vi "_BlankServer.vi"() -> ()   [LabVIEW 2012]
uses:
  ServerSubs/MyState.ctl
  ServerSubs/ROSLog.ctl
  SubVIs/_ROSDirection.ctl
  SubVIs/_ROSControl.ctl
  ServerSubs/requestTopic.ctl
panel:
  out "Log of port":string
  out "Queue log":string
  out "Last Reply":string
  out "Registered topics":T1[](array[typedef])
  out "Registering":bool
  out "MyState":T3
  out "(Un)Reg Text":string
  out "Setup":string
  out "Cmd Log":T4[](array[typedef])
  out "Connections Error log":string
  out "Connections":T5(array[cluster])
  out "Error log":string
  in  "stop":bool
  in  "ROS":T1={"topic port"=1236, "Node"="/labview", "topic"="/robot/head/command_head_nod", "type"="std_msgs/Bool", "node port"=7000, "error "={"status"=FALSE, "code"=0, "source"=""}, "Direction"=enum."Publisher", "APIs"=[], "Update (ms)"=1, "write queue"=1}
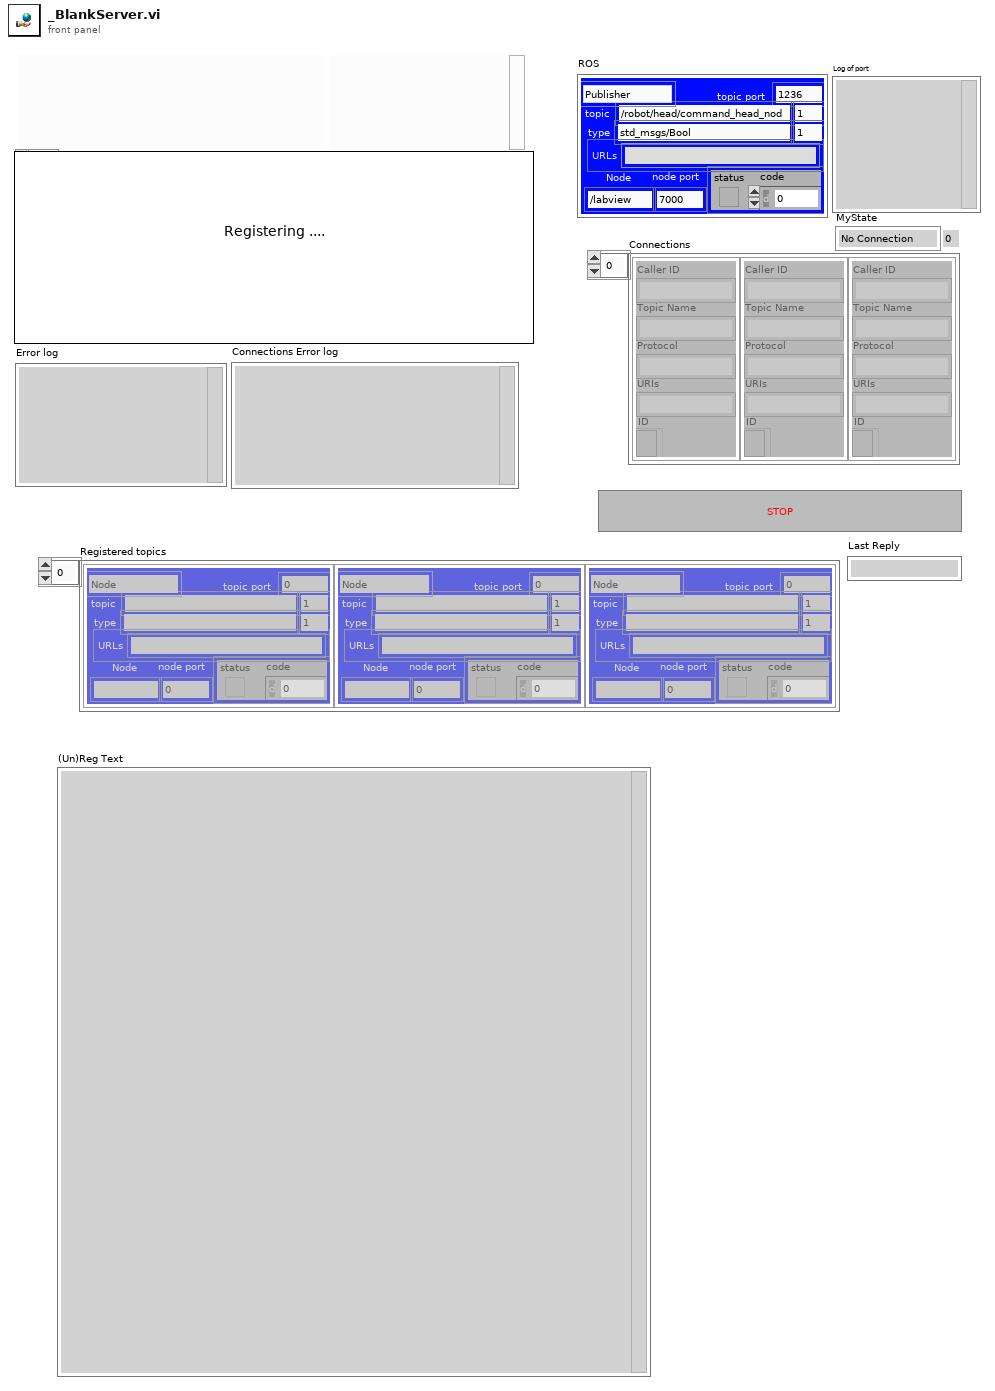
[diagram p1: front panel]
types:
  T1 = typedef "_ROSControl.ctl" = cluster{"topic port":u16, "Node":string, "topic":string, "type":string, "node port":u32, "error ":errorcluster, "Direction":T2, "APIs":string[], "Update (ms)":u16, "write queue":u16}
  T2 = typedef "_ROSDirection.ctl" = enum16{"Node", "Publisher", "Subscriber", "Service Client"}
  T3 = typedef "MyState.ctl" = enum16{"No Connection", "Registered", "Connected", "Close"}
  T4 = typedef "ROSLog.ctl" = cluster{"Sent":string, "Reply":string, "MethodName":string, "success":bool, "Dir1":string, "Dir2":string, "Time Stamp":string}
  T5 = cluster{"Caller ID":string, "Topic Name":string, "Protocol":string, "URIs":string, "ID":refnum<k5>}[]
  T6 = typedef "requestTopic.ctl" = cluster{"New Subscriber":cluster{"Caller ID":string, "Topic Name":string, "Protocol":string, "URIs":string, "ID":refnum<k5>}, "ROS of Server":T1, "new port":u16}
  T7 = cluster{"Code":i32, "Status Message":string, "APIs":string[]}
  T8 = cluster{"Caller ID":string, "Topic Name":string, "Protocol":string, "URIs":string, "ID":refnum<k5>}
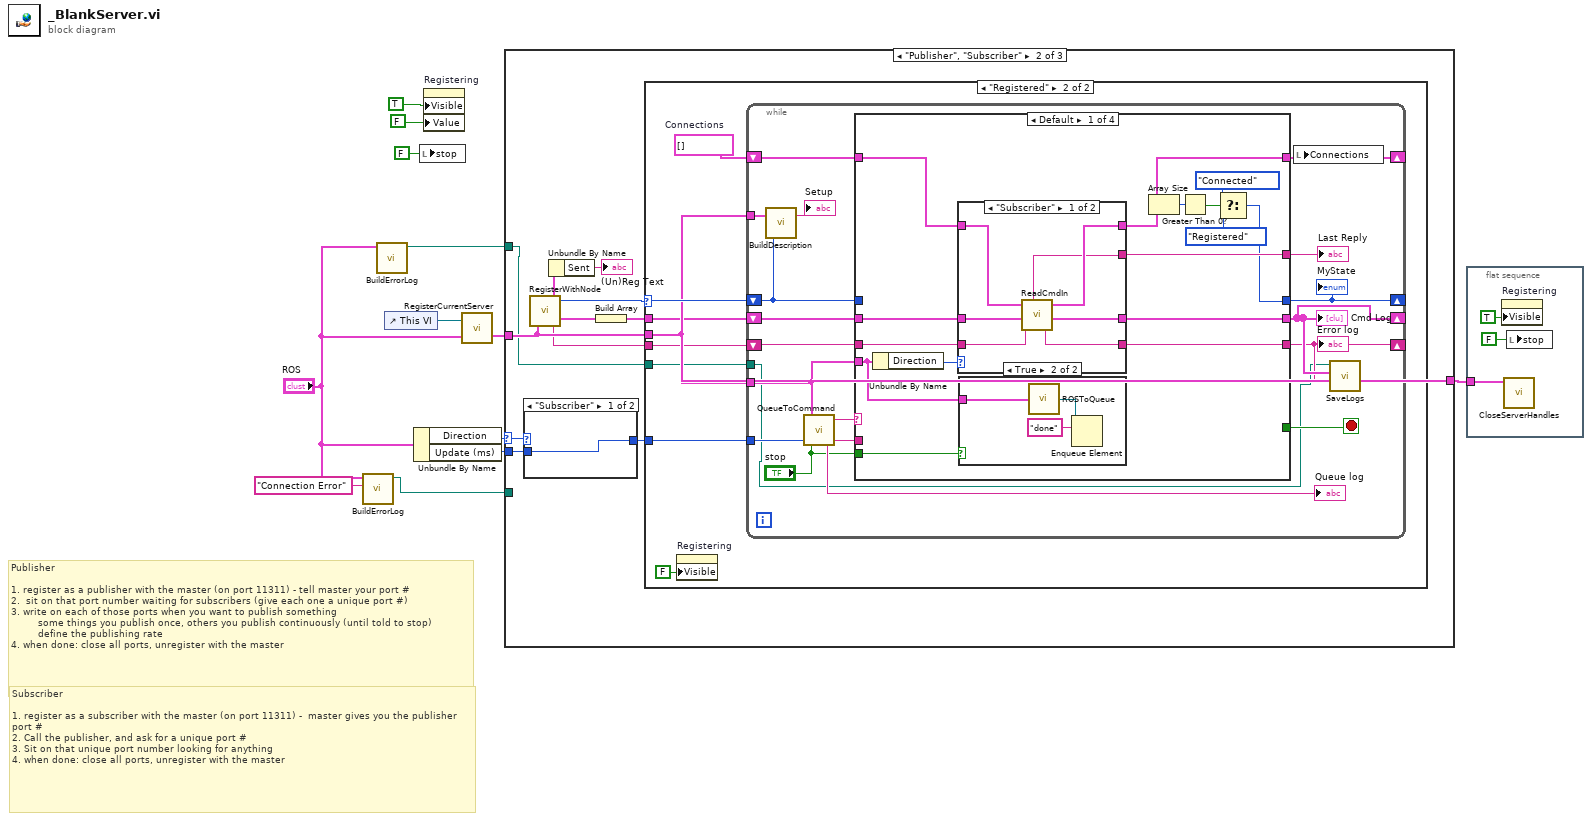
[diagram p0: block diagram]
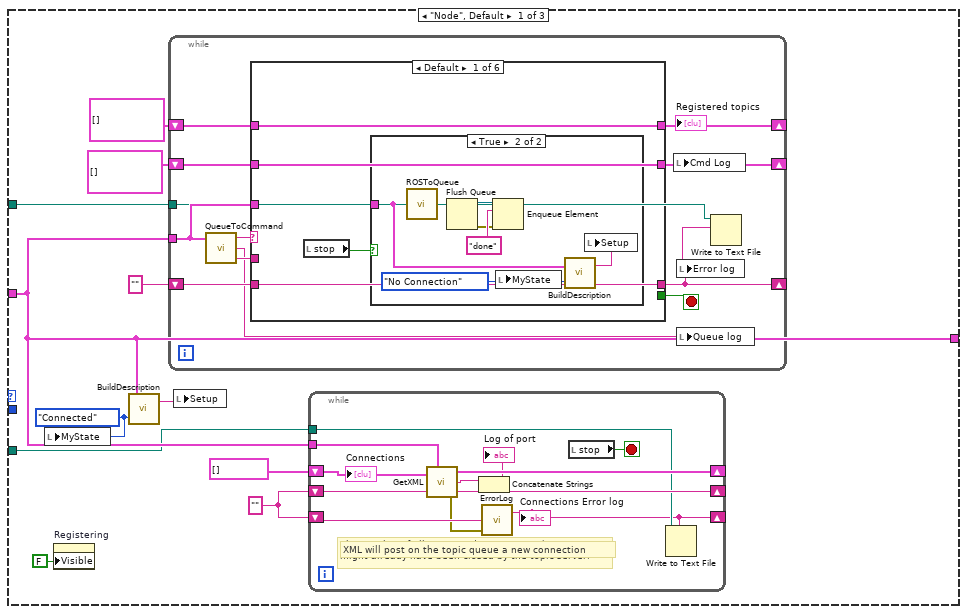
[diagram p2: hidden frame]
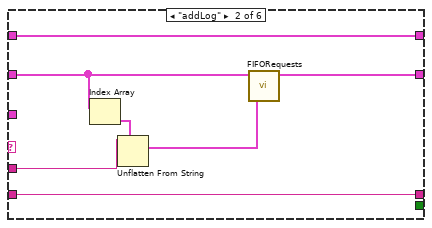
[diagram p4: hidden frame]
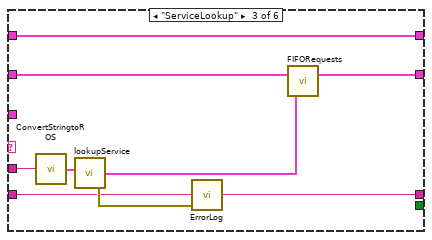
[diagram p5: hidden frame]
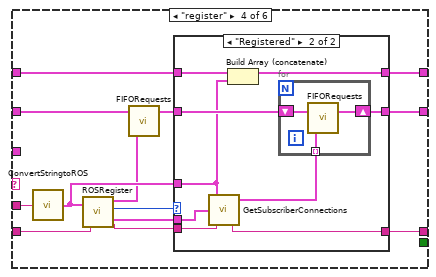
[diagram p6: hidden frame]
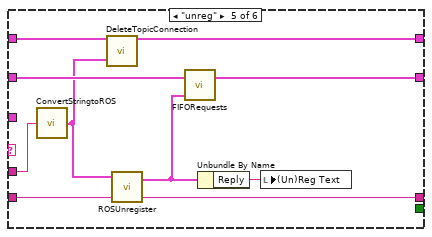
[diagram p8: hidden frame]
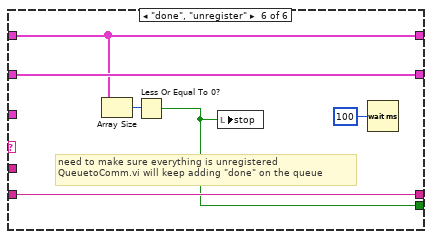
[diagram p9: hidden frame]
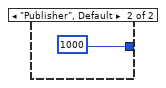
[diagram p10: hidden frame]
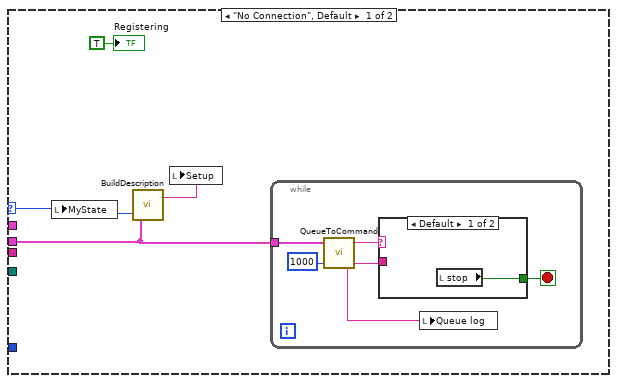
[diagram p11: hidden frame]
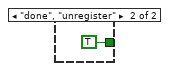
[diagram p12: hidden frame]
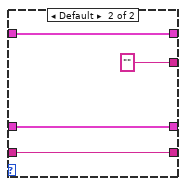
[diagram p13: hidden frame]
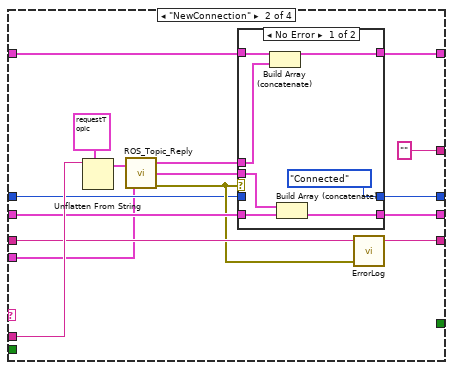
[diagram p15: hidden frame]
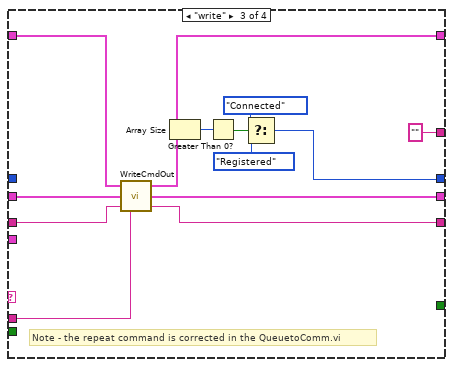
[diagram p17: hidden frame]
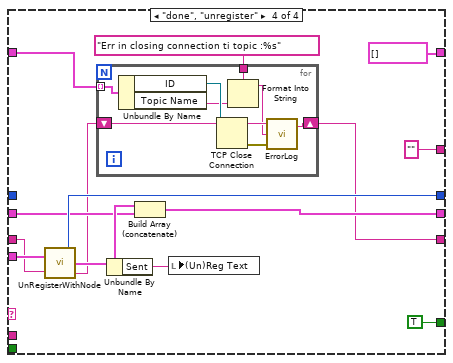
[diagram p18: hidden frame]
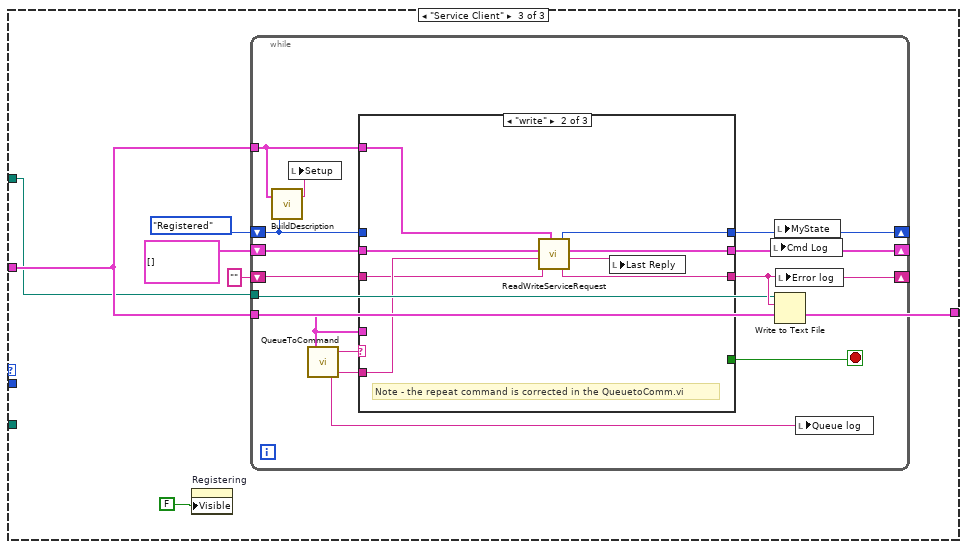
[diagram p19: hidden frame]
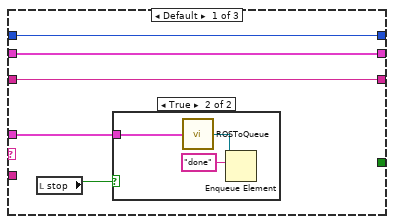
[diagram p20: hidden frame]
diagram:
  # "Subscriber\n\n1. register as a subscriber with the master (on port 11311) -  master gives you the publisher port #\n2. Call the publisher, and ask for a unique port #\n3. Sit on that unique port number looking for anything\n4. when done: close all ports, unregister with the master"
  # "Publisher\n\n1. register as a publisher with the master (on port 11311) - tell master your port #\n2.  sit on that port number waiting for subscribers (give each one a unique port #)\n3. write on each of those ports when you want to publish something\n         some things you publish once, others you publish continuously (until told to stop)\n         define the publishing rate\n4. when done: close all ports, unregister with the master"
  n1 = call "BuildErrorLog.vi"("Error Type"="Connection Error", "ROS"="ROS") -> ("error log path"=w1:path)  [unwired: 9 in]
  n2 = call "BuildErrorLog.vi"("ROS"="ROS") -> ("error log path"=w4:path)  [unwired: 10 in]
  n3 = control-ref of="This VI"() -> (w7:refnum<vi>)
  n4 = Unbundle By Name("ROS") -> ("Direction"=w10:T2, "Update (ms)"=w5:u16)
  n5 = local write "stop"(FALSE ("stop")) -> ()
  n6 = property on="Registering" class="Bool (strict)"("Visible"=TRUE ("Registering"), "Value"=FALSE ("Registering")) -> ()  [unwired: 2 in, 2 out]
  n7 = call "RegisterCurrentServer.vi"("ROS in"="ROS", "This VI"=w7) -> ("ROS out"=w6:T1)  [unwired: 1 in]
  n8 = case shown="\"Publisher\", \"Subscriber\"" w10 {
    selector: w10 -> [_ w125 _]
    tunnel: w6 -> [w17 w128 w265]
    tunnel: [w17 w128 w265] -> w8
    tunnel: w5 -> [_ w120 _]
    tunnel: w4 -> [w14 w119 w260]
    tunnel: w1 -> [w13 _ _]
    frame "Node", Default {
      w16 = "" ("String out")
      w21 = MyState."Connected" ("MyState")
      n9 = local write "MyState"(w21) -> ()
      n10 = property on="Registering" class="Bool (strict)"("Visible"=FALSE ("Registering")) -> ()  [unwired: 2 in, 2 out]
      n11 = call "BuildDescription.vi"("MyState"=w21, "ROS in"=w17) -> ("Setup"=w22:string)  [unwired: 1 in]
      n12 = while {
        shift-right: [w25] -> _
        shift-left: "" ("String out") -> [w34]
        shift-right: [w33] -> _
        shift-left: T4[] [] ("Requests Out") -> [w32]
        shift-right: [w31] -> _
        shift-left: T1[] [] -> [w30]
        tunnel: w17 -> [w26]
        tunnel: w14 -> [w24]
        stop <- w35 stop-if-true
        n13 = call "QueueToCommand.vi"("ROS"=w26) -> ("data"=w28:string, "Queue log"=w27:string, "Command"=w29:string)  [unwired: 2 in]
        n14 = case shown="Default" w29 {
          tunnel: [_ _ _ _ _ w103] -> w35
          tunnel: w28 -> [_ w52 w62 w76 w101 _]
          tunnel: w34 -> [w40 w54 w59 w75 w100 w107]
          tunnel: [w40 w54 w58 w64 w99 w107] -> w25
          tunnel: [w39 w48 w55 w74 w96 w106] -> w33
          tunnel: w32 -> [w39 w49 w56 w67 w97 w106]
          tunnel: [w38 w53 w63 w72 w93 w105] -> w31
          tunnel: w30 -> [w38 w53 w63 w73 w94 w105]
          tunnel: w26 -> [w36 _ _ _ _ _]
          frame Default {
            n15 = local read "stop"() -> (w37:bool)
            n16 = case shown="True" w37 {
              tunnel: w36 -> [_ w42]
              frame False {
              }
              frame True {
                w43 = MyState."No Connection" ("MyState")
                n17 = call "ROSToQueue.vi"("ROS"=w42) -> ("queue"=w45:refnum<queue>)  [unwired: 3 in, 1 out]
                n18 = Flush Queue(queue=w45) -> (queue out=w41:refnum<queue>, error out=w46:errorcluster)  [unwired: 1 in, 1 out]
                n19 = Enqueue Element(queue=w41, element="done" ("regular expression"), error in (no error)=w46) -> ()  [unwired: 1 in, 3 out]
                n20 = local write "MyState"(w43) -> ()
                n21 = call "BuildDescription.vi"("MyState"=w43, "ROS in"=w42) -> ("Setup"=w44:string)  [unwired: 1 in]
                n22 = local write "Setup"(w44) -> ()
              }
            }
          }
          frame "addLog" {
            n23 = Index Array(array=w49) -> (element=w51:T4)  [unwired: 1 in]
            n24 = Unflatten From String(type=w51, binary string=w52) -> (value=w50:T4)  [unwired: 3 in, 2 out]
            n25 = call "FIFORequests.vi"("Log"=w50, "Requests in"=w49) -> ("Requests out"=w48:T4[])  [unwired: 1 in]
          }
          frame "ServiceLookup" {
            n26 = call "ConvertStringtoROS.vi"("string in"=w62) -> ("ROS"=w61:T1)
            n27 = call "lookupService.vi"("Service ROS"=w61) -> ("error out"=w60:errorcluster, "Log"=w57:T4)  [unwired: 3 in]
            n28 = call "ErrorLog.vi"("error in"=w60, "String in"=w59) -> ("String out"=w58:string)  [unwired: 1 in, 1 out]
            n29 = call "FIFORequests.vi"("Log"=w57, "Requests in"=w56) -> ("Requests out"=w55:T4[])  [unwired: 1 in]
          }
          frame "register" {
            n30 = call "ConvertStringtoROS.vi"("string in"=w76) -> ("ROS"=w71:T1)
            n31 = call "ROSRegister.vi"("Err In"=w75, "ROS to register"=w71) -> ("Err Out"=w65:string, "Response"=w70:T7, "MyState"=w69:T3, "Log"=w68:T4)
            n32 = call "FIFORequests.vi"("Log"=w68, "Requests in"=w67) -> ("Requests out"=w66:T4[])  [unwired: 1 in]
            n33 = case shown="\"Registered\"" w69 {
              tunnel: w66 -> [w78 w88]
              tunnel: [w78 w87] -> w74
              tunnel: w73 -> [w79 w86]
              tunnel: [w79 w85] -> w72
              tunnel: w71 -> [_ w83]
              tunnel: w70 -> [_ w82]
              tunnel: w65 -> [w77 w81]
              tunnel: [w77 w80] -> w64
              frame Default {
              }
              frame "Registered" {
                n34 = call "GetSubscriberConnections.vi"("Err in"=w81, "Response"=w82, "ROS registered"=w83) -> ("Err out"=w80:string, "Logs out"=w84:T4[])  [unwired: 1 out]
                n35 = Build Array (concatenate)(w86, w83) -> (w85:T1[])
                n36 = for {
                  tunnel: w84 -> [w89] mode=indexing
                  shift-right: [w90] -> w87
                  shift-left: w88 -> [w91]
                  n37 = call "FIFORequests.vi"("Log"=w89, "Requests in"=w91) -> ("Requests out"=w90:T4[])  [unwired: 1 in]
                }
              }
            }
          }
          frame "unreg" {
            n38 = call "ConvertStringtoROS.vi"("string in"=w101) -> ("ROS"=w92:T1)
            n39 = call "DeleteTopicConnection.vi"("ROS"=w92, "Con In"=w94) -> ("Con out"=w93:T1[])
            n40 = call "ROSUnregister.vi"("Err in"=w100, "Server ROS"=w92) -> ("Err out"=w99:string, "Log"=w95:T4)  [unwired: 1 in]
            n41 = call "FIFORequests.vi"("Log"=w95, "Requests in"=w97) -> ("Requests out"=w96:T4[])  [unwired: 1 in]
            n42 = Unbundle By Name(w95) -> ("Reply"=w98:string)
            n43 = local write "(Un)Reg Text"(w98) -> ()
          }
          frame "done", "unregister" {
            # "need to make sure everything is unregistered\nQueuetoComm.vi will keep adding \"done\" on the queue"
            n44 = Array Size(array=w105) -> (size(s)=w104:i32)
            n45 = Less Or Equal To 0?(x=w104) -> (x <= 0?=w103:bool)
            n46 = local write "stop"(w103) -> ()
            n47 = Wait (ms)(milliseconds to wait=u32 100) -> ()  [unwired: 1 out]
          }
        }
        "Registered topics" <- w31
        n48 = local write "Cmd Log"(w33) -> ()
        n49 = local write "Error log"(w25) -> ()
        n50 = local write "Queue log"(w27) -> ()
        n51 = Write to Text File(file (use dialog)=w24, text=w25) -> ()  [unwired: 2 in, 3 out]
      }
      n52 = local write "Setup"(w22) -> ()
      n53 = while {
        shift-right: [w118] -> _
        shift-left: T5 [] ("Subscribers") -> [w110]
        tunnel: w17 -> [w116]
        shift-right: [w108] -> _
        shift-left: w16 -> [w117]
        shift-right: [w111] -> _
        shift-left: w16 -> [w113]
        tunnel: w13 -> [w109]
        stop <- w114 stop-if-true
        # "This is a log of all requested connections (some\nmight already have been closed by the topic server)"
        # "XML will post on the topic queue a new connection"
        n54 = call "GetXML.vi"("Node ROS"=w116, "Subscribers in"=w110) -> ("error IO"=w115:errorcluster, "reply"=w112:string, "Subscribers Out"=w118:T5)
        n55 = Concatenate Strings(w112, w113) -> (w111:string)
        "Log of port" <- w111
        n56 = call "ErrorLog.vi"("error in"=w115, "String in"=w117) -> ("String out"=w108:string)  [unwired: 1 in, 1 out]
        "Connections Error log" <- w108
        n57 = local read "stop"() -> (w114:bool)
        n58 = Write to Text File(file (use dialog)=w109, text=w108) -> ()  [unwired: 2 in, 3 out]
        "Connections" <- w110
      }
    }
    frame "Publisher", "Subscriber" {
      n59 = case shown="\"Subscriber\"" w125 {
        tunnel: [w129 1000 ("timeout in ms (1000)")] -> w124
        tunnel: w120 -> [w129 _]
        frame "Subscriber" {
        }
        frame "Publisher", Default {
        }
      }
      n60 = call "RegisterWithNode.vi"("ROS"=w128) -> ("MyState"=w126:T3, "Log"=w123:T4, "Error"=w121:string)
      n61 = Unbundle By Name(w123) -> ("Sent"=→"(Un)Reg Text":string)
      n62 = Build Array(w123) -> (w122:T4[])
      n63 = case shown="\"Registered\"" w126 {
        selector: w126 -> [w133 w149]
        tunnel: w128 -> [w131 w147]
        tunnel: w124 -> [_ w146]
        tunnel: w122 -> [_ w145]
        tunnel: w121 -> [_ w144]
        tunnel: w119 -> [_ w143]
        frame "No Connection", Default {
          n64 = local write "MyState"(w133) -> ()
          n65 = call "BuildDescription.vi"("MyState"=w133, "ROS in"=w131) -> ("Setup"=w134:string)  [unwired: 1 in]
          n66 = local write "Setup"(w134) -> ()
          n67 = while {
            tunnel: w131 -> [w135]
            stop <- w140 stop-if-true
            n68 = call "QueueToCommand.vi"("timeout"=1000 ("timeout in ms (-1)"), "ROS"=w135) -> ("data"=w139:string, "Queue log"=w136:string, "Command"=w137:string)  [unwired: 1 in]
            n69 = case shown="Default" w137 {
              tunnel: [w141 TRUE] -> w140
              tunnel: w139 -> [_ _]
              frame Default {
                n70 = local read "stop"() -> (w141:bool)
              }
              frame "done", "unregister" {
              }
            }
            n71 = local write "Queue log"(w136) -> ()
          }
          "Registering" <- TRUE ("Registering")
        }
        frame "Registered" {
          w150 = T5 []  # Connections
          n72 = property on="Registering" class="Bool (strict)"("Visible"=FALSE ("Registering")) -> ()  [unwired: 2 in, 2 out]
          n73 = while {
            shift-right: [w152] -> _
            shift-left: w144 -> [w169]
            shift-right: [w166] -> _
            shift-left: w145 -> [w167]
            shift-right: [w164] -> _
            shift-left: w149 -> [w155]
            tunnel: w147 -> [w163]
            tunnel: w147 -> [w154]
            shift-right: [w157] -> _
            shift-left: w150 -> [w162]
            tunnel: w146 -> [w156]
            tunnel: w143 -> [w151]
            stop <- w161 stop-if-true
            n74 = call "BuildDescription.vi"("MyState"=w155, "ROS in"=w163) -> ("Setup"=→"Setup":string)  [unwired: 1 in]
            n75 = call "QueueToCommand.vi"("timeout"=w156, "Stop Btn Pressed?"="stop", "ROS"=w154) -> ("data"=w168:string, "Queue log"=→"Queue log":string, "Command"=w159:string)
            n76 = case shown="Default" w159 {
              tunnel: [w182 w204 w237 w243] -> w152
              tunnel: w169 -> [w181 w205 w236 w240]
              tunnel: [w173 w202 w227 w251] -> w164
              tunnel: w168 -> [_ w210 w233 _]
              tunnel: w167 -> [w180 w208 w235 w246]
              tunnel: [w183 w207 w234 w245] -> w166
              tunnel: w162 -> [w179 w214 w231 w244]
              tunnel: [w174 w213 w225 T5 [] ("Connections Out")] -> w157
              tunnel: [_ _ _ TRUE] -> w161
              tunnel: [w184 "" ("String out") "" ("String out") "" ("String out")] -> w160
              tunnel: w155 -> [_ w201 _ _]
              tunnel: w154 -> [w171 w199 _ w241]
              tunnel: "stop" -> [w170 _ _ _]
              frame Default {
                n77 = Unbundle By Name(w171) -> ("Direction"=w172:T2)
                n78 = case shown="\"Subscriber\"" w172 {
                  tunnel: [w186 "" ("String out")] -> w184
                  tunnel: [w191 w192] -> w174
                  tunnel: [w190 w194] -> w183
                  tunnel: [w189 w193] -> w182
                  tunnel: w181 -> [w188 w193]
                  tunnel: w180 -> [w187 w194]
                  tunnel: w179 -> [w185 w192]
                  frame "Subscriber" {
                    n79 = call "ReadCmdIn.vi"("Connections"=w185, "Log in"=w187, "Err in"=w188) -> ("data"=w186:string, "Connections out"=w191:T5, "Log out"=w190:T4[], "Err out"=w189:string)  [unwired: 1 in]
                  }
                  frame Default {
                  }
                }
                n80 = case shown="True" w170 {
                  tunnel: w171 -> [_ w196]
                  frame False {
                  }
                  frame True {
                    n81 = call "ROSToQueue.vi"("ROS"=w196) -> ("queue"=w197:refnum<queue>)  [unwired: 3 in, 1 out]
                    n82 = Enqueue Element(queue=w197, element="done") -> ()  [unwired: 2 in, 3 out]
                  }
                }
                n83 = Array Size(array=w174) -> (size(s)=w178:i32)
                n84 = Greater Than 0?(x=w178) -> (x > 0?=w175:bool)
                n85 = Select(t=MyState."Connected" ("f"), s=w175, f=MyState."Registered") -> (s? t:f=w173:T3)
              }
              frame "NewConnection" {
                n86 = Unflatten From String(type=T6 {"New Subscriber"={"Caller ID"="", "Topic Name"="", "Protocol"="", "URIs"="", "ID"=refnum}, "ROS of Server"={"topic port"=0, "Node"="", "topic"="", "type"="", "node port"=0, "error "={"status"=FALSE, "code"=0, "source"=""}, "Direction"=enum."Node", "APIs"=[], "Update (ms)"=0, "write queue"=0}, "new port"=0} ("data"), binary string=w210) -> (value=w206:T6)  [unwired: 3 in, 2 out]
                n87 = call "ROS_Topic_Reply.vi"("data"=w206, "My ROS"=w199) -> ("Subscriber out"=w211:T8, "Log"=w209:T4, "error IO"=w203:errorcluster)
                n88 = case shown="No Error" w203 {
                  tunnel: w214 -> [w221 w224]
                  tunnel: [w220 w224] -> w213
                  tunnel: w211 -> [w219 _]
                  tunnel: w209 -> [w218 _]
                  tunnel: w208 -> [w217 w223]
                  tunnel: [w216 w223] -> w207
                  tunnel: [MyState."Connected" ("MyState") w222] -> w202
                  tunnel: w201 -> [_ w222]
                  frame No Error {
                    n89 = Build Array (concatenate)(w221, w219) -> (w220:T5)
                    n90 = Build Array (concatenate)(w218, w217) -> (w216:T4[])
                  }
                  frame Error {
                  }
                }
                n91 = call "ErrorLog.vi"("error in"=w203, "Error String"=w205) -> ("String out"=w204:string)  [unwired: 1 in, 1 out]
              }
              frame "write" {
                # "Note - the repeat command is corrected in the QueuetoComm.vi"
                n92 = call "WriteCmdOut.vi"("Connections In"=w231, "Log in"=w235, "Err in"=w236, "data"=w233) -> ("Connections Out"=w225:T5, "Log out"=w234:T4[], "Err out"=w237:string)  [unwired: 1 in]
                n93 = Array Size(array=w225) -> (size(s)=w226:i32)
                n94 = Greater Than 0?(x=w226) -> (x > 0?=w230:bool)
                n95 = Select(t=MyState."Connected" ("f"), s=w230, f=MyState."Registered") -> (s? t:f=w227:T3)
              }
              frame "done", "unregister" {
                n96 = call "UnRegisterWithNode.vi"("ROS"=w241, "Err in"=w240) -> ("MyState"=w251:T3, "Log"=w247:T4, "Err out"=w239:string)
                n97 = for {
                  tunnel: w244 -> [w259] mode=indexing
                  shift-right: [w257] -> w243
                  shift-left: w239 -> [w256]
                  tunnel: "Err in closing connection ti topic :%s" ("String in") -> [w254]
                  n98 = Unbundle By Name(w259) -> ("ID"=w258:refnum<k5>, "Topic Name"=w253:string)
                  n99 = TCP Close Connection(connection ID=w258) -> (error out=w255:errorcluster)  [unwired: 2 in, 1 out]
                  n100 = Format Into String(format string=w254, w253) -> (resulting string=w252:string)  [unwired: 2 in, 1 out]
                  n101 = call "ErrorLog.vi"("error in"=w255, "String in"=w252, "Error String"=w256) -> ("String out"=w257:string)  [unwired: 1 out]
                }
                n102 = Unbundle By Name(w247) -> ("Sent"=w250:string)
                n103 = Build Array (concatenate)(w247, w246) -> (w245:T4[])
                n104 = local write "(Un)Reg Text"(w250) -> ()
              }
            }
            "Cmd Log" <- w166
            "MyState" <- w164
            "Last Reply" <- w160
            n105 = local write "Connections"(w157) -> ()
            n106 = call "SaveLogs.vi"("Err in"=w152, "Cmd log"=w166, "error log path"=w151) -> ()  [unwired: 9 in]
          }
        }
      }
    }
    frame "Service Client" {
      n107 = property on="Registering" class="Bool (strict)"("Visible"=FALSE ("Registering")) -> ()  [unwired: 2 in, 2 out]
      n108 = while {
        shift-right: [w267] -> _
        shift-left: "" ("String out") -> [w279]
        shift-right: [w272] -> _
        shift-left: T4[] [] ("Log") -> [w277]
        shift-right: [w273] -> _
        shift-left: MyState."Registered" ("MyState") -> [w276]
        tunnel: w265 -> [w269]
        tunnel: w265 -> [w268]
        tunnel: w260 -> [w266]
        stop <- w275 stop-if-true
        n109 = call "BuildDescription.vi"("MyState"=w276, "ROS in"=w269) -> ("Setup"=w270:string)  [unwired: 1 in]
        n110 = local write "Setup"(w270) -> ()
        n111 = call "QueueToCommand.vi"("ROS"=w268) -> ("data"=w278:string, "Queue log"=w271:string, "Command"=w274:string)  [unwired: 2 in]
        n112 = case shown="\"write\"" w274 {
          tunnel: [w281 w289 w298] -> w267
          tunnel: w279 -> [w281 w290 w298]
          tunnel: [w283 w293 MyState."No Connection" ("MyState")] -> w273
          tunnel: w278 -> [_ w291 _]
          tunnel: w277 -> [w282 w295 w299]
          tunnel: [w282 w294 w299] -> w272
          tunnel: w276 -> [w283 _ _]
          tunnel: [_ _ TRUE] -> w275
          tunnel: w269 -> [_ w292 _]
          tunnel: w268 -> [w280 _ _]
          frame Default {
            n113 = local read "stop"() -> (w284:bool)
            n114 = case shown="True" w284 {
              tunnel: w280 -> [_ w285]
              frame False {
              }
              frame True {
                n115 = call "ROSToQueue.vi"("ROS"=w285) -> ("queue"=w286:refnum<queue>)  [unwired: 3 in, 1 out]
                n116 = Enqueue Element(queue=w286, element="done") -> ()  [unwired: 2 in, 3 out]
              }
            }
          }
          frame "write" {
            # "Note - the repeat command is corrected in the QueuetoComm.vi"
            n117 = call "ReadWriteServiceRequest.vi"("Service ROS"=w292, "Error in"=w290, "data"=w291, "Log in"=w295) -> ("Error out"=w289:string, "String Read"=w288:string, "Log"=w294:T4[], "MyState"=w293:T3)  [unwired: 1 in]
            n118 = local write "Last Reply"(w288) -> ()
          }
          frame "done", "unregister" {
            # "stop all repeating connections"
          }
        }
        n119 = local write "Cmd Log"(w272) -> ()
        n120 = local write "MyState"(w273) -> ()
        n121 = Write to Text File(file (use dialog)=w266, text=w267) -> ()  [unwired: 2 in, 3 out]
        n122 = local write "Error log"(w267) -> ()
        n123 = local write "Queue log"(w271) -> ()
      }
    }
  }
  n124 = flat-sequence {
    tunnel: w8 -> [w300]
    frame #0 {
      n125 = property on="Registering" class="Bool (strict)"("Visible"=TRUE ("Registering")) -> ()  [unwired: 2 in, 2 out]
      n126 = call "CloseServerHandles.vi"("ROS"=w300) -> ()
      n127 = local write "stop"(FALSE ("stop")) -> ()
    }
  }
